vi "Operaciones con Strings.vi"() -> ()   [LabVIEW 2022 SP3]
panel:
  out "Thermometer 3":dbl(slide) scale=0.0..100.0
  out "Thermometer 2":dbl(slide) scale=0.0..100.0 scale format="%#_6f"
  out "Thermometer":dbl(slide) scale=0.0..100.0
  out "TERCER DATO 3":string
  out "SEGUNDO DATO 2":string
  out "PRIMER DATO 2":string
  in  "Datos Rx HARDWARE 2":string
  out "Palabra invertida":string
  out "first char last":string
  out "TEXTO RESULTADO 3":string caption="Result"
  out "TEXTO RESULTADO 2":string caption="Result"
  in  "TEXTO INICIAL 2":string caption="Beginning Text"
  in  "TEXTO INICIAL":string caption="Beginning Text"
  out "TEXTO RESULTADO":string caption="Result"
  out "RESIDUO":string
  out "match substring":string
  out "SGUNDO DATO":string
  out "RESIDUO":string
  out "CARACTER SEPARADOR":string
  out "PRIMER DATO":string
  in  "Datos Rx HARDWARE":string
  out "Palabra buscada y remplazada":string
  out "Palabra Remplazada":string
  out "Remplazo de string":string
  in  "tamaño del texto":i32
  in  "offset (0)":i32
  out "Extraccion de string":string
  out "TAMAÑO 2 PALABRA CONCATENADA":i32
  out "INDICADOR CONCATENADO":string
  in  "CONTROL STRING 2":string
  out "TAMAÑO":i32
  out "INDICADOR":string
  in  "CONTROL STRING":string
  # "Teoria"
  # "Ejercicios"
  # "Ejemplo 1: DATO ADQUIRIDO"
  # "SENSOR1,SENSOR2,SENSOR3F : 50.32,45.334,12.879F"
  # "BUILT TEXT  EXPRESS VI"
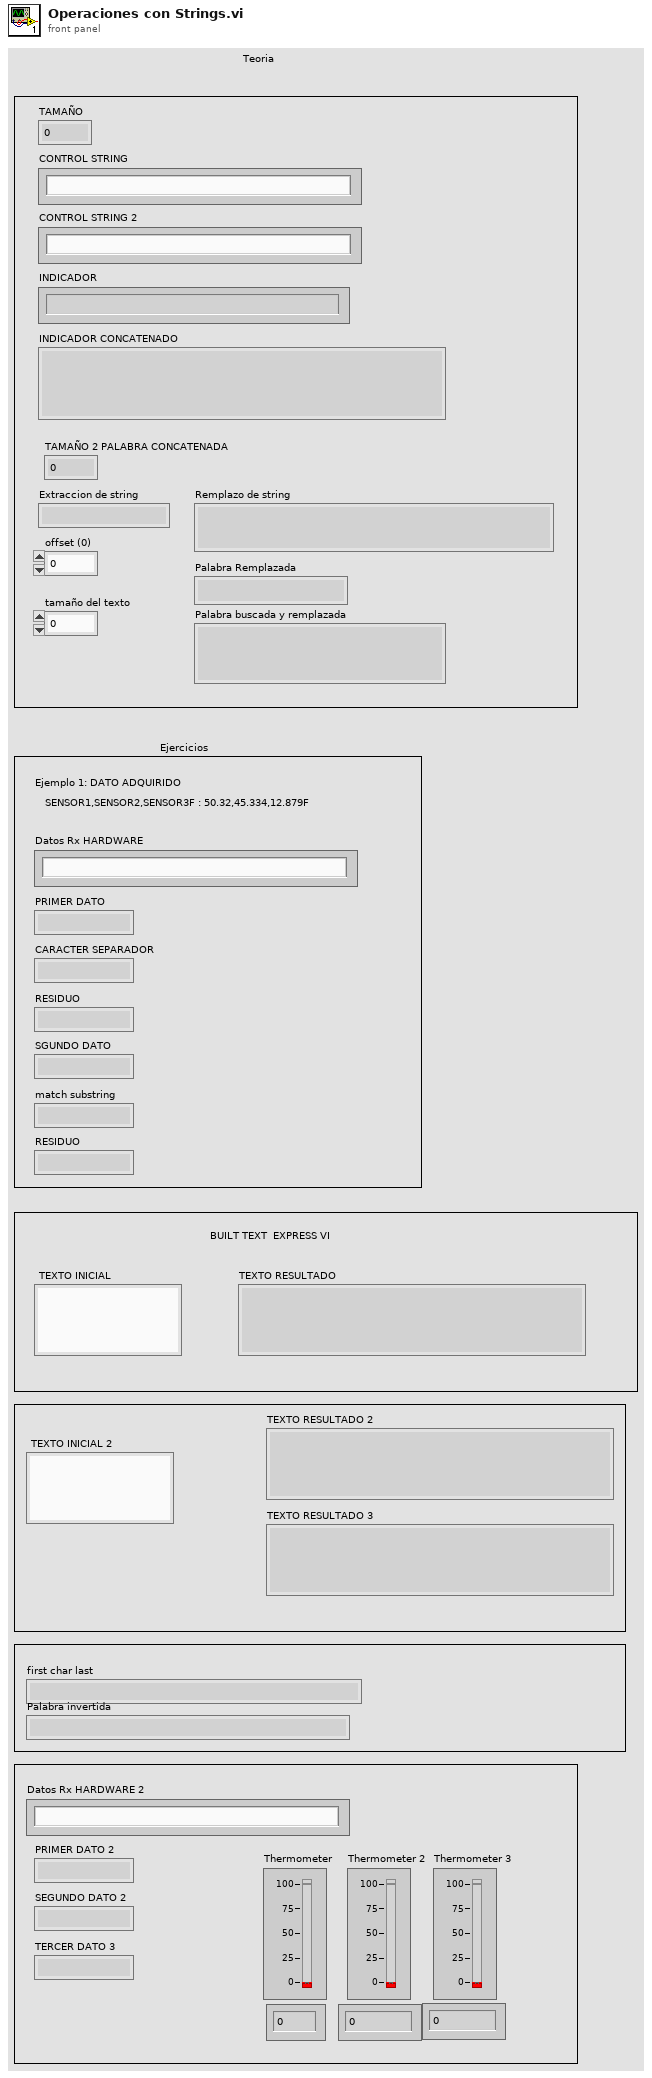
[diagram p1: front panel]
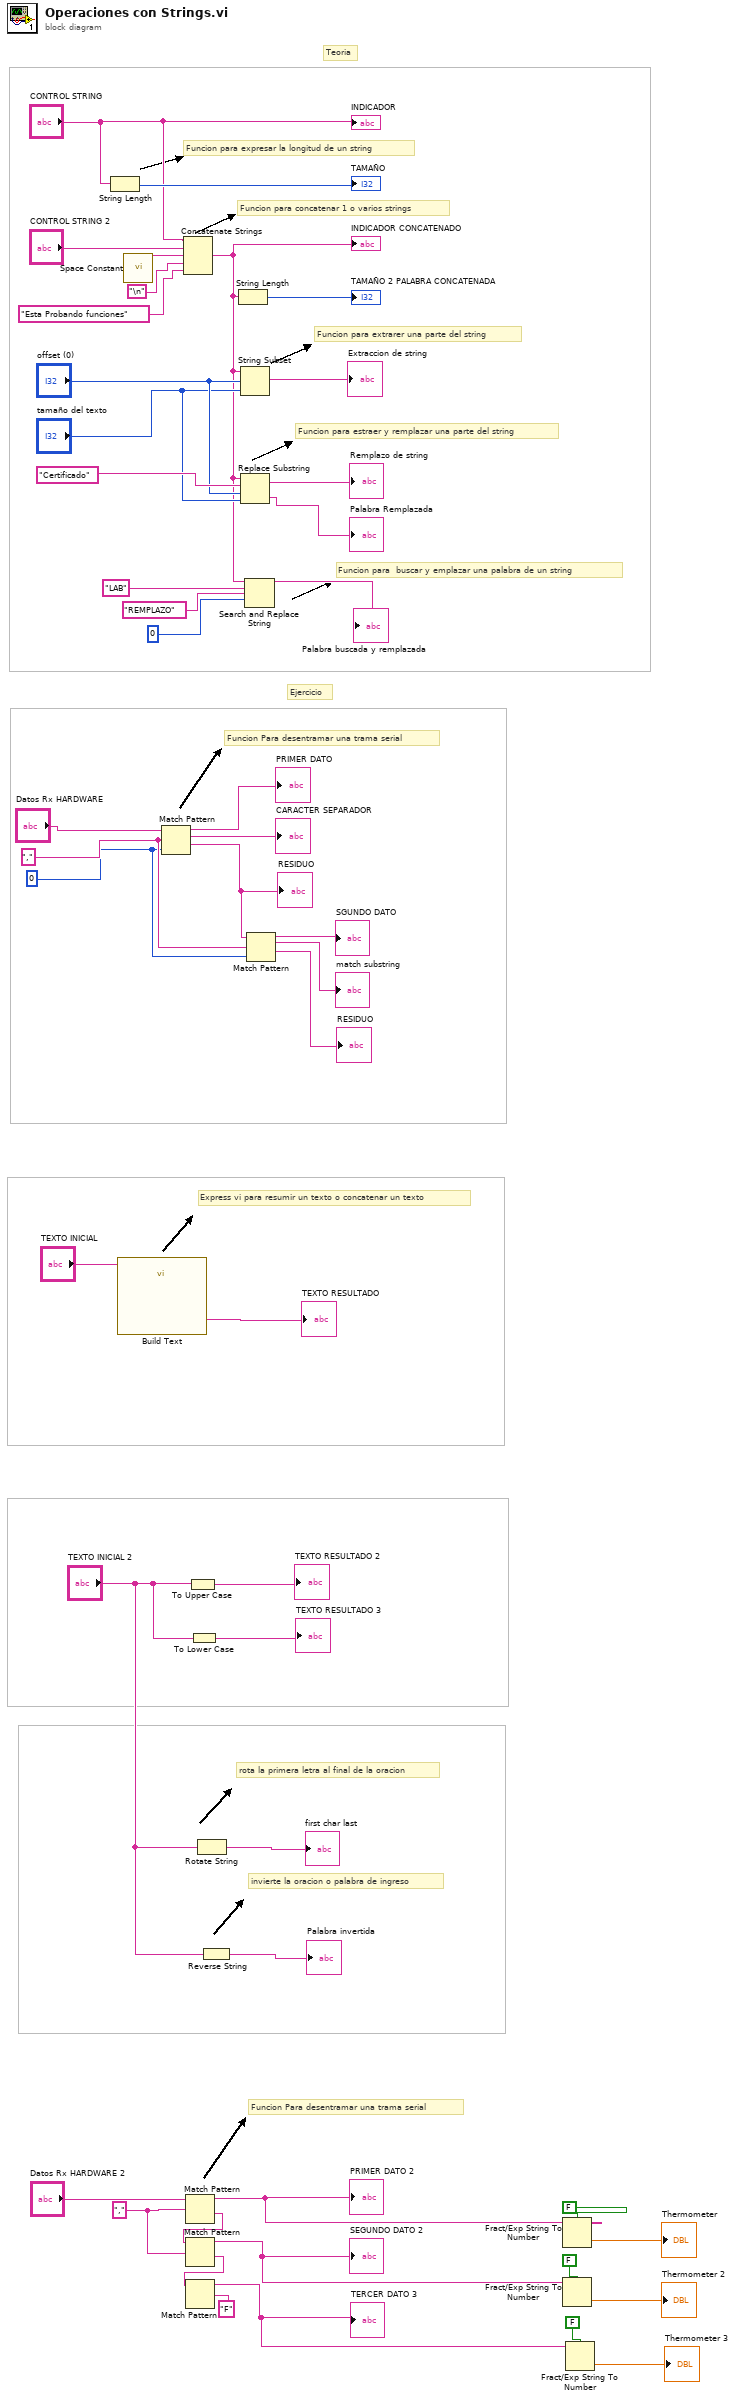
[diagram p0: block diagram]
diagram:
  w3 = "," ("regular expression")
  w25 = 0 ("offset (0)")
  w26 = "," ("regular expression")
  # "Funcion Para desentramar una trama serial"
  # "invierte la oracion o palabra de ingreso"
  # "rota la primera letra al final de la oracion"
  # "Express vi para resumir un texto o concatenar un texto"
  # "Funcion Para desentramar una trama serial"
  # "Ejercicio"
  # "Teoria"
  # "Funcion para  buscar y emplazar una palabra de un string"
  # "Funcion para estraer y remplazar una parte del string"
  # "Funcion para extrarer una parte del string"
  # "Funcion para concatenar 1 o varios strings"
  # "Funcion para expresar la longitud de un string"
  n1 = String Length(string="CONTROL STRING") -> (length=→"TAMAÑO":i32)
  n2 = call "Build Text"("Beginning Text"="TEXTO INICIAL") -> ("Result"=→"TEXTO RESULTADO":string)  [unwired: 13 in, 1 out]
  n3 = call <vilib>:"Space Constant.vi"() -> ("String"=w44:string)
  n4 = Match Pattern(string="Datos Rx HARDWARE", regular expression=w26, offset (0)=w25) -> (before substring=→"PRIMER DATO":string, match substring=→"CARACTER SEPARADOR":string, after substring=w27:string)  [unwired: 1 out]
  "RESIDUO" <- w27
  n5 = Concatenate Strings("CONTROL STRING", "CONTROL STRING 2", w44, "\n", "Esta Probando funciones") -> (w36:string)
  "INDICADOR CONCATENADO" <- w36
  n6 = Match Pattern(string="Datos Rx HARDWARE 2", regular expression=w3) -> (before substring=w9:string, after substring=w13:string)  [unwired: 1 in, 2 out]
  "PRIMER DATO 2" <- w9
  n7 = Match Pattern(string=w13, regular expression=w3) -> (before substring=w2:string, after substring=w6:string)  [unwired: 1 in, 2 out]
  "SEGUNDO DATO 2" <- w2
  n8 = Match Pattern(string=w6, regular expression="F") -> (before substring=w1:string)  [unwired: 1 in, 3 out]
  "TERCER DATO 3" <- w1
  n9 = To Upper Case(1:"TEXTO INICIAL 2") -> (0:→"TEXTO RESULTADO 2":string)
  n10 = To Lower Case(string="TEXTO INICIAL 2") -> (all lower case string=→"TEXTO RESULTADO 3":string)
  n11 = Rotate String(1:"TEXTO INICIAL 2") -> (0:→"first char last":string)
  n12 = Reverse String(1:"TEXTO INICIAL 2") -> (0:→"Palabra invertida":string)
  n13 = String Length(string=w36) -> (length=→"TAMAÑO 2 PALABRA CONCATENADA":i32)
  n14 = String Subset(string=w36, offset (0)="offset (0)", length (rest)="tamaño del texto") -> (substring=→"Extraccion de string":string)
  n15 = Replace Substring(2:"tamaño del texto", 3:"offset (0)", 4:"Certificado", 5:w36) -> (0:→"Palabra Remplazada":string, 1:→"Remplazo de string":string)
  n16 = Search and Replace String(input string=w36, search string="LAB", replace string="REMPLAZO" ("replace string (\"\")"), offset=0 ("offset (0)")) -> (result string=→"Palabra buscada y remplazada":string)  [unwired: 4 in, 3 out]
  n17 = Match Pattern(string=w27, regular expression=w26, offset (0)=w25) -> (before substring=→"SGUNDO DATO":string, match substring=→"match substring":string, after substring=→"RESIDUO":string)  [unwired: 1 out]
  n18 = Fract/Exp String To Number(use system decimal point (T)=FALSE, string=w9) -> (number=→"Thermometer":dbl)  [unwired: 2 in, 1 out]
  n19 = Fract/Exp String To Number(use system decimal point (T)=FALSE, string=w2) -> (number=→"Thermometer 2":dbl)  [unwired: 2 in, 1 out]
  n20 = Fract/Exp String To Number(use system decimal point (T)=FALSE, string=w1) -> (number=→"Thermometer 3":dbl)  [unwired: 2 in, 1 out]
  "INDICADOR" <- "CONTROL STRING"
